vi "心音分析.vi"() -> ()   [LabVIEW 2018]
uses:
  <vilib>/Analysis/3filter.llb/Filter Passband Type.ctl
  <vilib>/Analysis/4window.llb/windowTd.ctl
  <vilib>/Analysis/3filter.llb/Butterworth Filter (DBL).vi
  <vilib>/express/express analysis/Spectral/Block/exnSpectralBlock spectral measurements RMS poly.vi
  <vilib>/express/express analysis/Spectral/Block/exnSpectralBlock spectral measurements RMS WFM.vi
  <vilib>/Analysis/3filter.llb/FIR Windowed Filter (DBL).vi
  <vilib>/Analysis/3filter.llb/Elliptic Filter (DBL).vi
  <vilib>/Analysis/3filter.llb/Chebyshev Filter (DBL).vi
  <vilib>/express/express analysis/Spectral/XNode/ExpressSpectralMeasurementsBlockNode.xnode
  <vilib>/Analysis/NI_AALBase.lvlib
  <vilib>/Analysis/NI_AALPro.lvlib
panel:
  in  "滤波器种类":u16(ring) caption="下拉列表" items=["FIR滤波器", "椭圆滤波器", "巴特沃斯滤波器", "切比雪夫滤波器"]
  in  "?":bool
  out "滤波后波形图":dbl[](graph)
  out "滤波后频谱":cluster{"f0":dbl, "df":dbl, "magnitude":dbl[]}(graph)
  out "加噪音后频谱":cluster{"f0":dbl, "df":dbl, "magnitude":dbl[]}(graph)
  out "心音频谱":cluster{"f0":dbl, "df":dbl, "magnitude":dbl[]}(graph)
  out "心音波形图":dbl[](graph)
  in  "路径":path
  in  "window":T1 caption="窗" items=["矩形"=0, "Hanning"=1, "Hamming"=2, "Blackman-Harris"=3, "Exact Blackman"=4, "Blackman"=5, "Flat Top"=6, "4阶Blackman-Harris "=7, "7阶Blackman-Harris"=8, "Low Sidelobe"=9, "Blackman Nuttall"=11, "三角"=30, "Bartlett-Hanning"=31, "Bohman"=32, "Parzen"=33, "Welch"=34, "Kaiser"=60, "Dolph-Chebyshev"=61, "高斯"=62]
  in  "停止":bool
  in  "滤波器阶数":i32
  in  "filter type":T2 caption="通带类型"
  in  "低频截止频率":dbl(slide) scale=0.0..500.0
  out "加噪音后波形图":dbl[](graph)
  in  "taps":i32=25 caption="抽头" min=1
  in  "采样数":i32=-128 caption="采样"
  in  "噪声幅值":dbl=1.0 format="%0.2f"
  # "基于LabVIEW的心音信号频域分析系统"
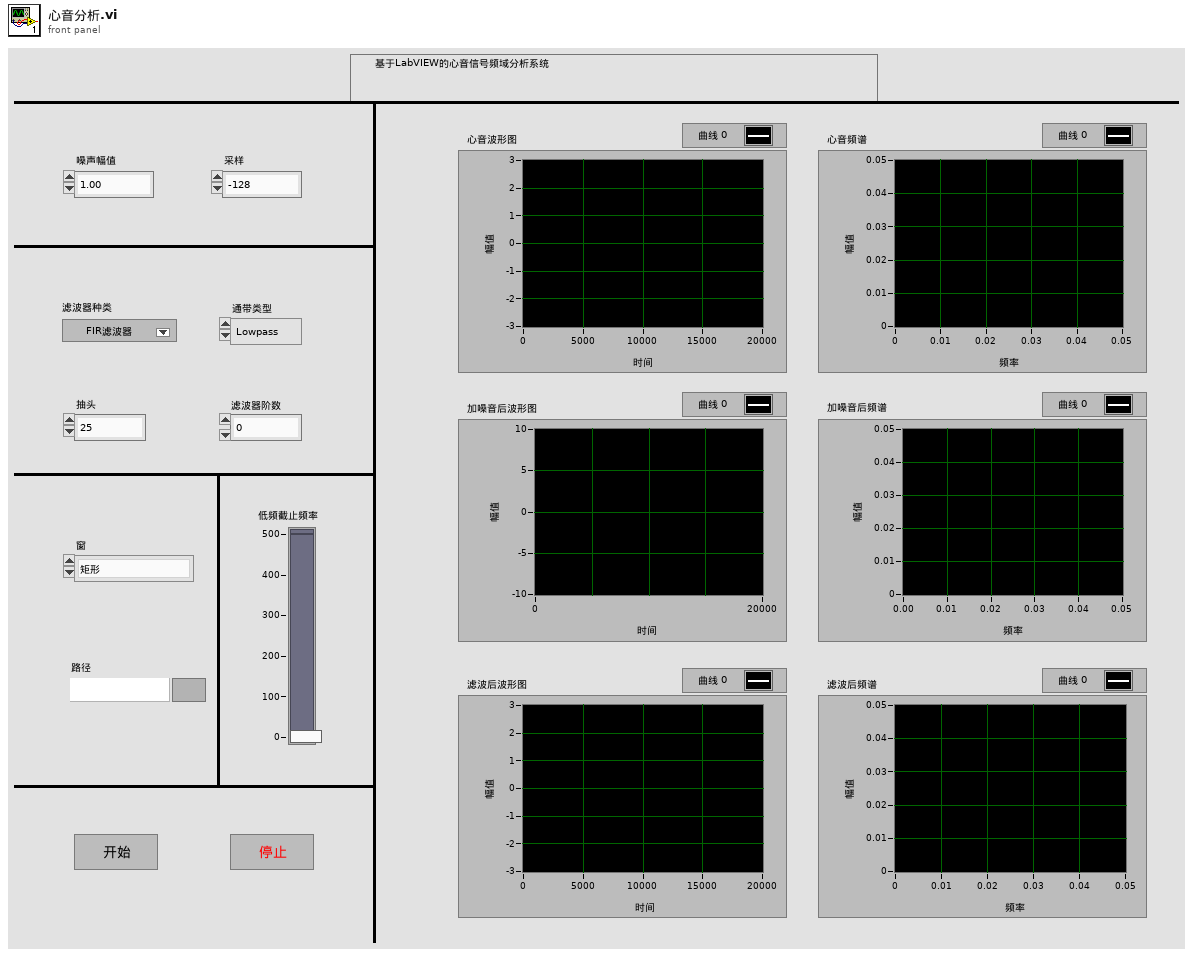
[diagram p1: front panel]
types:
  T1 = typedef "NI_AALPro.lvlib/windowTd.ctl" = u32
  T2 = typedef "NI_AALBase.lvlib/Filter Passband Type.ctl" = enum32{"Lowpass", "Highpass", "Bandpass", "Bandstop"}
  T3 = cluster{"averaging mode":u16, "weighting mode":u16, "number of averages":u32}
  T4 = cluster{"dB On (F)":bool, "unwrap phase (F)":bool, "convert to degree (F)":bool}
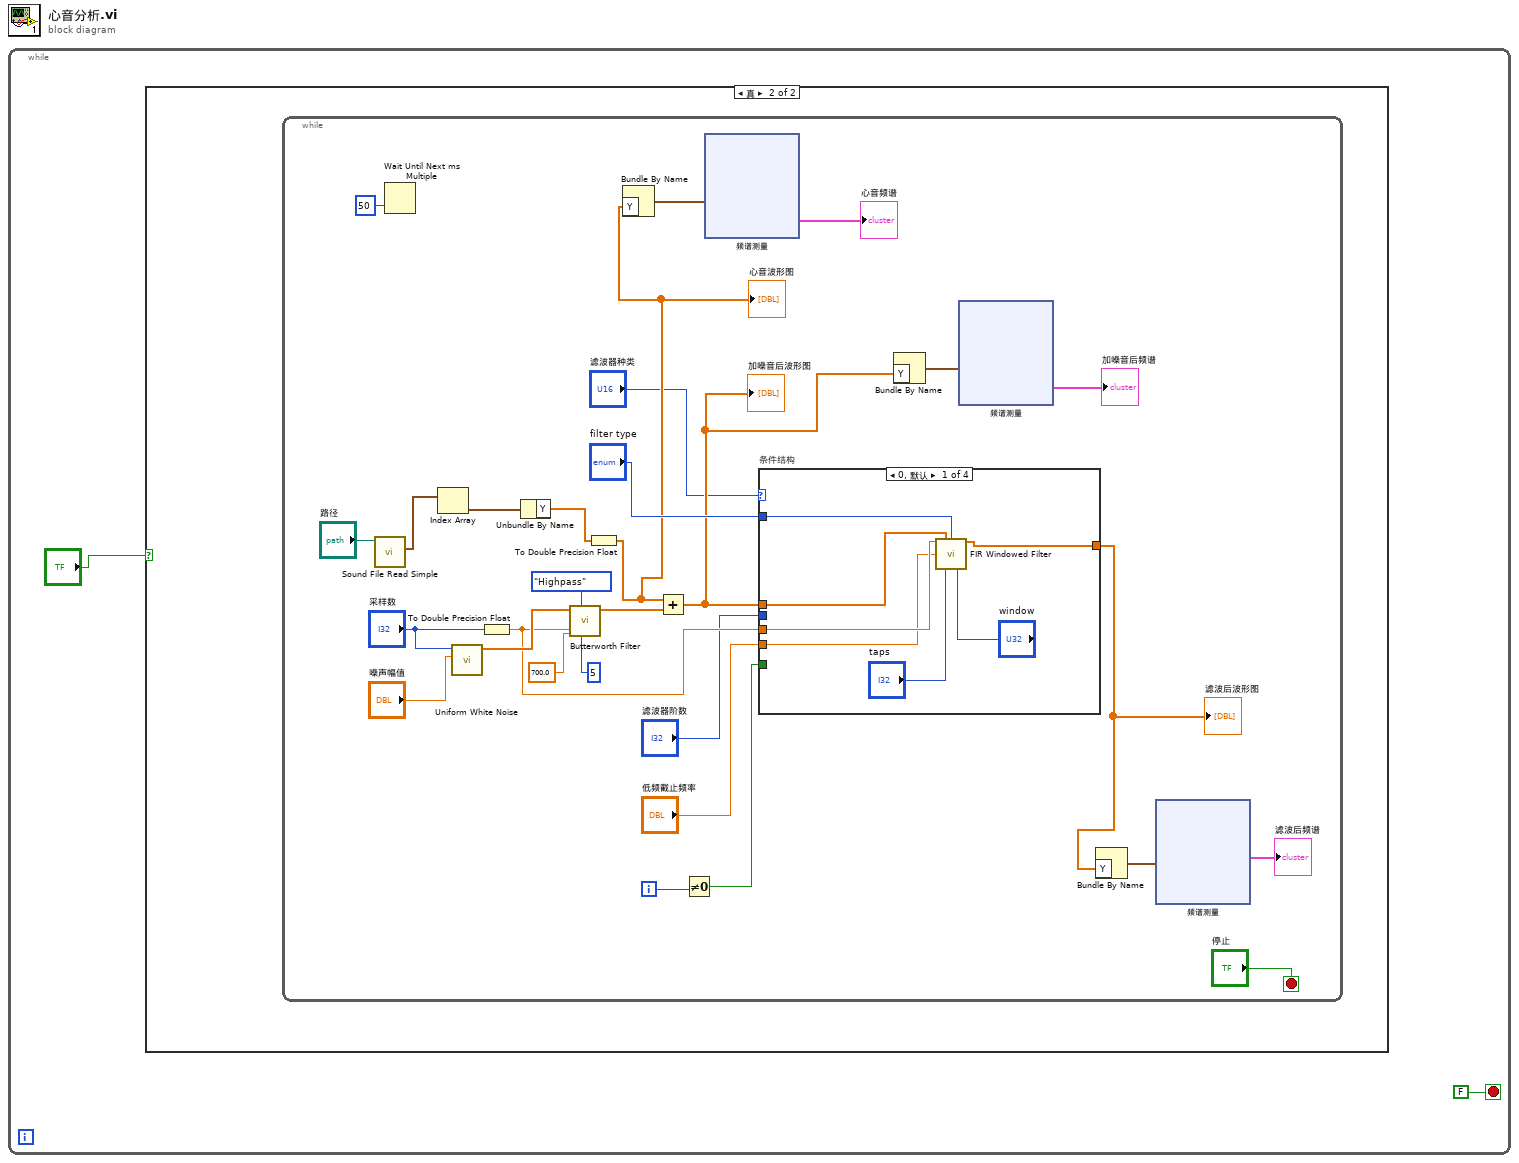
[diagram p0: block diagram]
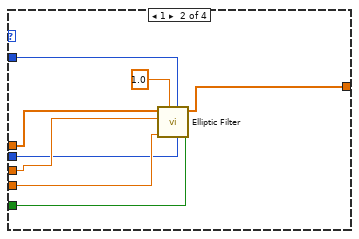
[diagram p3: hidden frame]
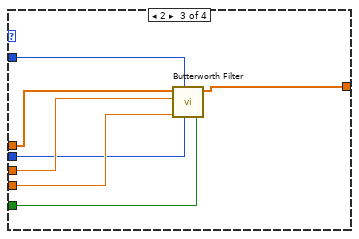
[diagram p4: hidden frame]
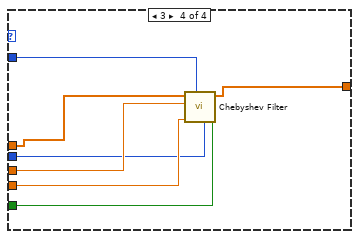
[diagram p5: hidden frame]
diagram:
  n1 = while {
    stop <- FALSE stop-if-true
    n2 = case shown="真" "?" {
      frame False {
      }
      frame True {
        n3 = while {
          i -> [w20]
          stop <- "停止" stop-if-true
          n4 = call <vilib>:"Sound File Read Simple.vi"("path"="路径") -> ("data"=w17:waveform(dbl)[])  [unwired: 7 in, 3 out]
          n5 = Wait Until Next ms Multiple(millisecond multiple=u32 50 ("毫秒倍数")) -> ()  [unwired: 1 out]
          n6 = Index Array(array=w17) -> (element=w16:waveform(dbl))  [unwired: 1 in]
          n7 = call <vilib>:"Uniform White Noise.vi"("amplitude"="噪声幅值", "samples"="采样数") -> ("uniform white noise"=w29:dbl[])  [unwired: 8 in, 1 out]
          n8 = To Double Precision Float(number="采样数") -> (double precision float=w26:dbl)
          n9 = Unbundle By Name(w16) -> ("Y"=w13:dbl[])
          n10 = call-poly <vilib>:"Butterworth Filter.vi"("order"=5, "filter type"=Filter_Passband_Type."Highpass", "low cutoff freq: fl"=700.0, "sampling freq: fs"=w26, "X"=w29) -> ("Filtered X"=w27:dbl[])  [unwired: 3 in, 1 out]
          n11 = To Double Precision Float(number=w13) -> (double precision float=w10:dbl[])
          "心音波形图" <- w10
          n12 = Bundle By Name("Y"=w10) -> (w9:waveform(dbl))  [unwired: 1 in]
          n13 = Add(x=w10, y=w27) -> (x+y=w12:dbl[])
          "加噪音后波形图" <- w12
          n14 = Not Equal To 0?(x=w20) -> (x != 0?=w22:bool)
          n15 = xnode "频谱测量"("信号"=w9) -> ("FFT - （均方根）"=→"心音频谱":cluster{"f0":dbl, "df":dbl, "magnitude":dbl[]})  [unwired: 1 in, 2 out]
          n16 = case "条件结构" shown="0, 默认" "滤波器种类" {
            tunnel: w12 -> [w66 w69 w82 w90]
            tunnel: w26 -> [w65 w75 w81 w89]
            tunnel: "低频截止频率" -> [w64 w76 w80 w88]
            tunnel: "filter type" -> [w67 w70 w77 w84]
            tunnel: "滤波器阶数" -> [_ w74 w78 w86]
            tunnel: w22 -> [_ w72 w79 w87]
            tunnel: [w63 w73 w83 w85] -> w6
            frame 0, Default {
              n17 = call-poly <vilib>:"FIR Windowed Filter.vi"("sampling freq: fs"=w65, "X"=w66, "filter type"=w67, "low cutoff freq: fl"=w64, "taps"="taps", "window"="window") -> ("Filtered X"=w63:dbl[])  [unwired: 8 in, 1 out]
            }
            frame 1 {
              n18 = call-poly <vilib>:"Elliptic Filter.vi"("init/cont (init:F)"=w72, "order"=w74, "filter type"=w70, "passband ripple (dB)"=1.0, "low cutoff freq: fl"=w76, "sampling freq: fs"=w75, "X"=w69) -> ("Filtered X"=w73:dbl[])  [unwired: 3 in, 1 out]
            }
            frame 2 {
              n19 = call-poly <vilib>:"Butterworth Filter.vi"("init/cont (init:F)"=w79, "order"=w78, "filter type"=w77, "low cutoff freq: fl"=w80, "sampling freq: fs"=w81, "X"=w82) -> ("Filtered X"=w83:dbl[])  [unwired: 2 in, 1 out]
            }
            frame 3 {
              n20 = call-poly <vilib>:"Chebyshev Filter.vi"("init/cont (init:F)"=w87, "order"=w86, "filter type"=w84, "low cutoff freq: fl"=w88, "sampling freq: fs"=w89, "X"=w90) -> ("Filtered X"=w85:dbl[])  [unwired: 4 in, 1 out]
            }
          }
          "滤波后波形图" <- w6
          n21 = Bundle By Name("Y"=w12) -> (w11:waveform(dbl))  [unwired: 1 in]
          n22 = xnode "频谱测量"("信号"=w11) -> ("FFT - （均方根）"=→"加噪音后频谱":cluster{"f0":dbl, "df":dbl, "magnitude":dbl[]})  [unwired: 1 in, 2 out]
          n23 = Bundle By Name("Y"=w6) -> (w8:waveform(dbl))  [unwired: 1 in]
          n24 = xnode "频谱测量"("信号"=w8) -> ("FFT - （均方根）"=→"滤波后频谱":cluster{"f0":dbl, "df":dbl, "magnitude":dbl[]})  [unwired: 1 in, 2 out]
        }
      }
    }
  }
